vi "Daq32-64WaitInId.vi"(6 "time(0.1)":i32=100, 8 "error in":errorcluster, 9 "Wait?":bool=TRUE, 10 "Status":bool, 11 "IO_Input":T1) -> (0 "error Out":errorcluster, 2 "TimeOut":bool, 3 "StatusOut":bool)   [LabVIEW 2015]
uses:
  global/InAndOutGB.vi
  global/IO_FlagGB.vi
  Ctrl/UniDaq_SelectInPut.ctl
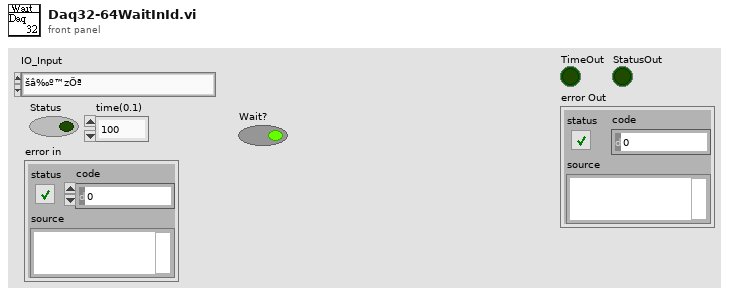
[diagram p1: front panel]
types:
  T1 = typedef "UniDaq_SelectInPut.ctl" = enum16{"šâ‰º™zÖª", "Ö÷ów™C¼Ü°²È«éT", "TF880有料", "TF300Ready", "TF300可吸料", "Îü×ìÒ»ÉÏÎ»™zÖª", "Îü×ìÒ»ÏÂÎ»™zÖª", "吸嘴一真空", "Îü×ì¶þÉÏÎ»™zÖª", "Îü×ì¶þÏÂÎ»™zÖª", "吸嘴二真空", "Îü×ìÈýÉÏÎ»™zÖª", "Îü×ìÈýÏÂÎ»™zÖª", "吸嘴三真空", "Îü×ìËÄÉÏÎ»™zÖª", "Îü×ìËÄÏÂÎ»™zÖª", "吸嘴四真空", "Ýd±P¿¿Î»é_Î»™zÖª", "Ýd±P¿¿Î»‰ºÎ»™zÖª", "²»Á¼Æ·ÁÏ±P™zÖª", "¾o¼±Í£Ö¹", "ÉÏÁÏ™C°²È«éT"}
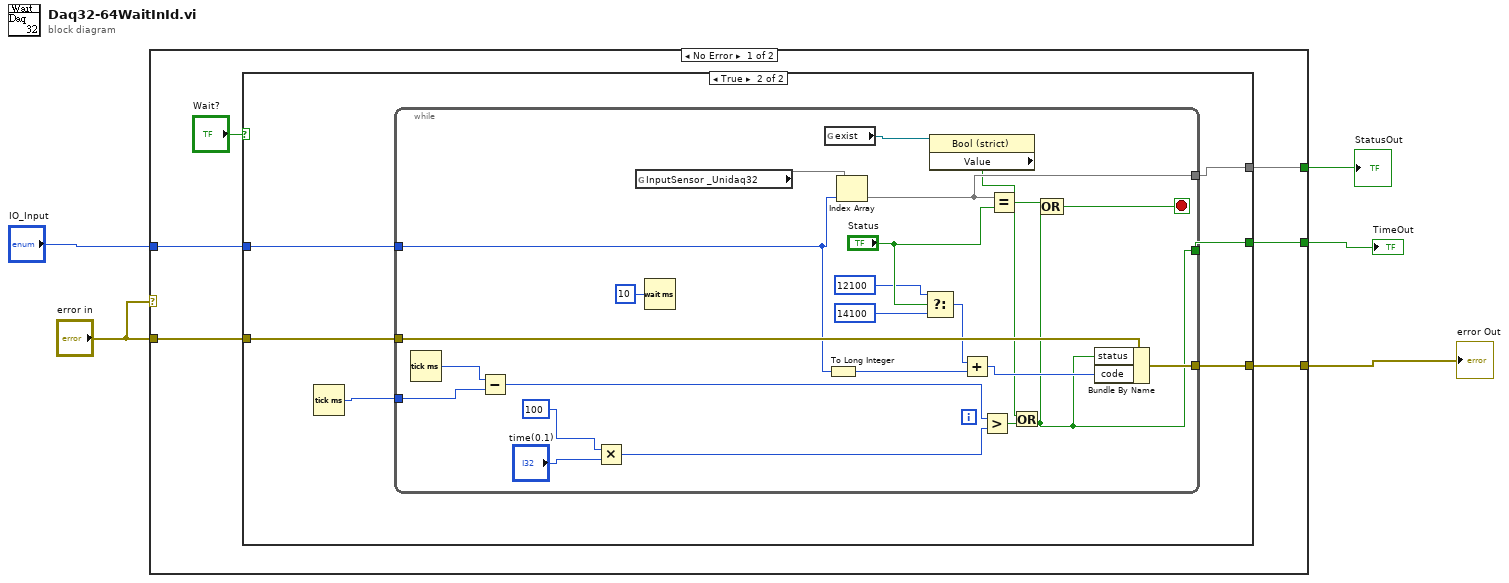
[diagram p0: block diagram]
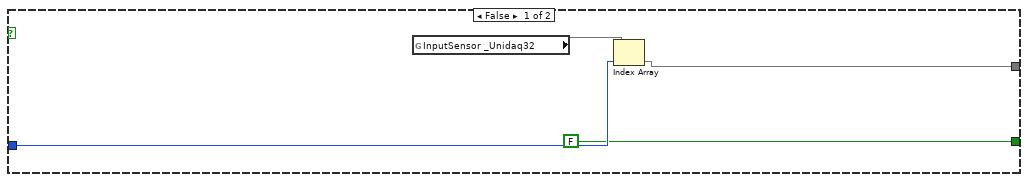
[diagram p2: hidden frame]
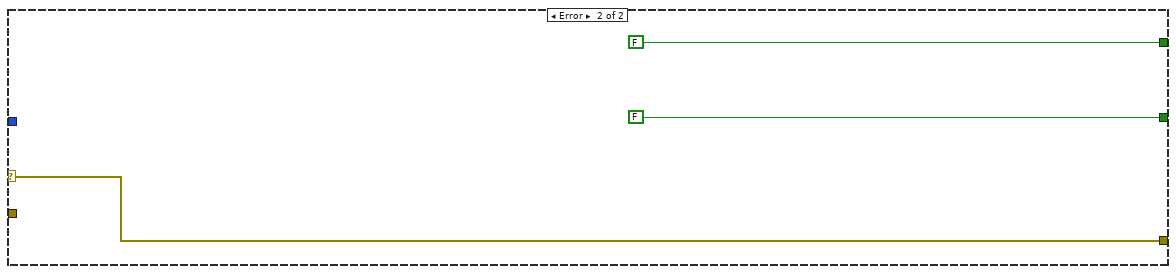
[diagram p3: hidden frame]
diagram:
  n1 = case shown="No Error" "error in" {
    selector: "error in" -> [_ w47]
    tunnel: [w11 FALSE] -> w5
    tunnel: "error in" -> [w10 _]
    tunnel: [w9 w47] -> w4
    tunnel: [w8 FALSE ("Boolean")] -> w2
    tunnel: "IO_Input" -> [w6 _]
    frame No Error {
      n2 = case shown="True" "Wait?" {
        tunnel: [FALSE w21] -> w11
        tunnel: w10 -> [_ w20]
        tunnel: [_ w19] -> w9
        tunnel: [w13 w18] -> w8
        tunnel: w6 -> [w14 w17]
        frame False {
          n3 = global read "InAndOutGB.vi" "InputSensor _Unidaq32"() -> (w15)
          n4 = Index Array(array=w15, index=w14) -> (element=w13)
        }
        frame True {
          n5 = Tick Count (ms)() -> (millisecond timer value=w16:u32)
          n6 = while {
            tunnel: [w33] -> w21
            tunnel: w20 -> [w42]
            tunnel: [w39] -> w19
            tunnel: [w32] -> w18
            tunnel: w17 -> [w30]
            tunnel: w16 -> [w27]
            stop <- w44 stop-if-true
            n7 = Tick Count (ms)() -> (millisecond timer value=w28:u32)
            n8 = Subtract(x=w28, y=w27) -> (x-y=w26:u32)
            n9 = Multiply(x=u32 100 ("milliseconds to wait"), y="time(0.1)") -> (x*y=w23:u32)
            n10 = global read "InAndOutGB.vi" "InputSensor _Unidaq32"() -> (w45)
            n11 = Wait (ms)(milliseconds to wait=u32 10) -> ()  [unwired: 1 out]
            n12 = global read "IO_FlagGB.vi" "exist"() -> (w29:refnum<vi>)
            n13 = To Long Integer(number=w30) -> (32bit integer=w34:i32)
            n14 = Index Array(array=w45, index=w30) -> (element=w32)
            n15 = Select(t=12100 ("y"), s="Status", f=14100 ("y")) -> (s? t:f=w35:i32)
            n16 = property class="Bool (strict)"(reference=w29) -> ("Value"=w31:bool)  [unwired: 1 in, 2 out]
            n17 = Add(x=w35, y=w34) -> (x+y=w40:i32)
            n18 = Greater?(x=w26, y=w23) -> (0:w41:bool)
            n19 = Equal?(x=w32, y="Status") -> (x = y?=w43:bool)
            n20 = Or(x=w31, y=w41) -> (x .or. y?=w33:bool)
            n21 = Compound Arithmetic op=OR(w43, w33) -> (w44:bool)
            n22 = Bundle By Name(cluster=w42, "status"=w33, "code"=w40) -> (w39:errorcluster)
          }
        }
      }
    }
    frame Error {
    }
  }
  "TimeOut" <- w5
  "error Out" <- w4
  "StatusOut" <- w2
